vi "SimulatedResult.vi"() -> (1 "MicPass?":bool, 2 "SPL":dbl, 3 "Pass?":bool)   [LabVIEW 2014]
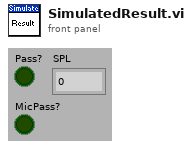
[diagram p1: front panel]
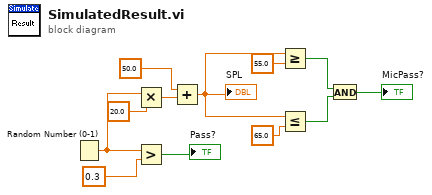
[diagram p0: block diagram]
diagram:
  n1 = Random Number (0-1)() -> (number: 0 to 1=w10:dbl)
  n2 = Multiply(x=w10, y=20.0) -> (x*y=w8:dbl)
  n3 = Greater?(x=w10, y=0.3) -> (0:→"Pass?":bool)
  n4 = Add(x=50.0 ("y"), y=w8) -> (x+y=w5:dbl)
  "SPL" <- w5
  n5 = Greater Or Equal?(x=w5, y=55.0) -> (x >= y?=w2:bool)
  n6 = Less Or Equal?(x=w5, y=65.0) -> (x <= y?=w3:bool)
  n7 = And(x=w2, y=w3) -> (x .and. y?=→"MicPass?":bool)
